vi "PH_PowerUnit_BaseClass.evt call Control Remote.vi"(0 "i ref in":refnum<vi>, 2 "PowerUnit":T1, 3 "Remote controlled?":bool, 5 "error in (no error)":errorcluster) -> (14 "i ref out":refnum<vi>, 19 "error out":errorcluster)   [LabVIEW 2014, in "PH_PowerUnit_BaseClass.lvlib"]
doc: "This VI sends the connected device the control remotelly command by a simple call."
uses:
  PH_PowerUnit_BaseClass.lvlib
  PH_PP_Common/PH_PP_Common.PUs.ctl
  CSCore/CSSystem/CoreLib/CoreLib.short 2 byte array.vi
  CSCore/CSSystem/CoreLib/CoreLib.lvlib
  CSCore/BaseProcess/BaseProcess.lvlib
  PH_PP_Common/PH_PP_Common.lvlib
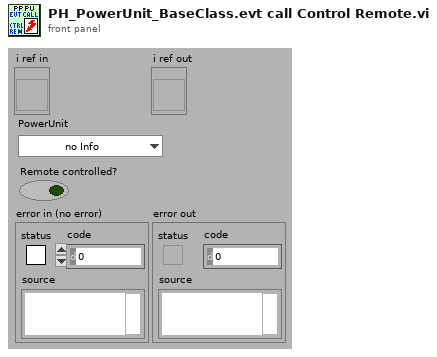
[diagram p1: front panel]
types:
  T1 = typedef "PH_PP_Common.lvlib/PH_PP_Common.PUs.ctl" = enum16{"no Info", "PA-19mm-1", "PA-19mm-2", "PA-45mm-PILC", "PA-45mm-MAIN", "MA-PU-1", "MA-PU-2", "MA-PU-3", "MA-PU-4", "MA-PU-5", "MA-PU-6", "MA-FR", "MA-PILC", "PA-45mm-DP"}
  T2 = typedef "CoreDefs.rawDataType.ctl" = i8[]
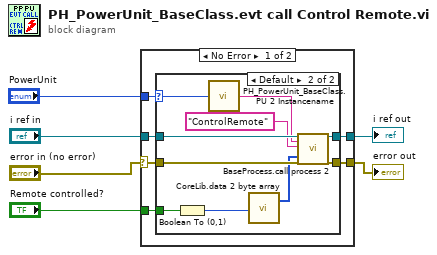
[diagram p0: block diagram]
diagram:
  n1 = case shown="No Error" "error in (no error)" {
    selector: "error in (no error)" -> [w8 w25]
    tunnel: [w12 w26] -> w2
    tunnel: [w11 w25] -> w3
    tunnel: "i ref in" -> [w10 w26]
    tunnel: "PowerUnit" -> [w9 _]
    tunnel: "Remote controlled?" -> [w7 _]
    frame No Error {
      n2 = case shown="Default" w9 {
        selector: w9 -> [_ w18]
        tunnel: [w14 w24] -> w12
        tunnel: [w13 w23] -> w11
        tunnel: w10 -> [w14 w22]
        tunnel: w8 -> [w13 w21]
        tunnel: w7 -> [_ w17]
        frame "no Info" {
        }
        frame Default {
          n3 = Boolean To (0,1)(Boolean=w17) -> (0, 1=w16:i16)
          n4 = call "PH_PowerUnit_BaseClass.PU 2 Instancename.vi"("PU"=w18) -> ("Instance Name"=w15:string)
          n5 = call-poly "CoreLib.data 2 byte array.vi"("i16"=w16) -> ("byteArray out"=w19:T2)  [unwired: 18 in]
          n6 = call "BaseProcess.call process 2.vi"("i ref in"=w22, "Object"=w15, "Selector"="ControlRemote", "Data"=w19, "error in (no error)"=w21) -> ("i ref out"=w24:refnum<vi>, "error out"=w23:errorcluster)  [unwired: 13 in]
        }
      }
    }
    frame Error {
    }
  }
  "error out" <- w3
  "i ref out" <- w2
